vi "Collect Data.vi"(6 "Vicon Logging Signal":dbl, 7 "Motor Command":dbl, 8 "Current Time (s)":dbl, 9 "rt fifo":refnum<k33>, 10 "Target Lossy Data":T2, 11 "Sensors":T1) -> ()   [LabVIEW 2018]
uses:
  Target Lossy Data.ctl
  Sensor Data.ctl
  Target Logging Cluster.ctl
  Logging Data Cluster.ctl
  Target Logging Control Signals.ctl
  Target Logging Sensors.ctl
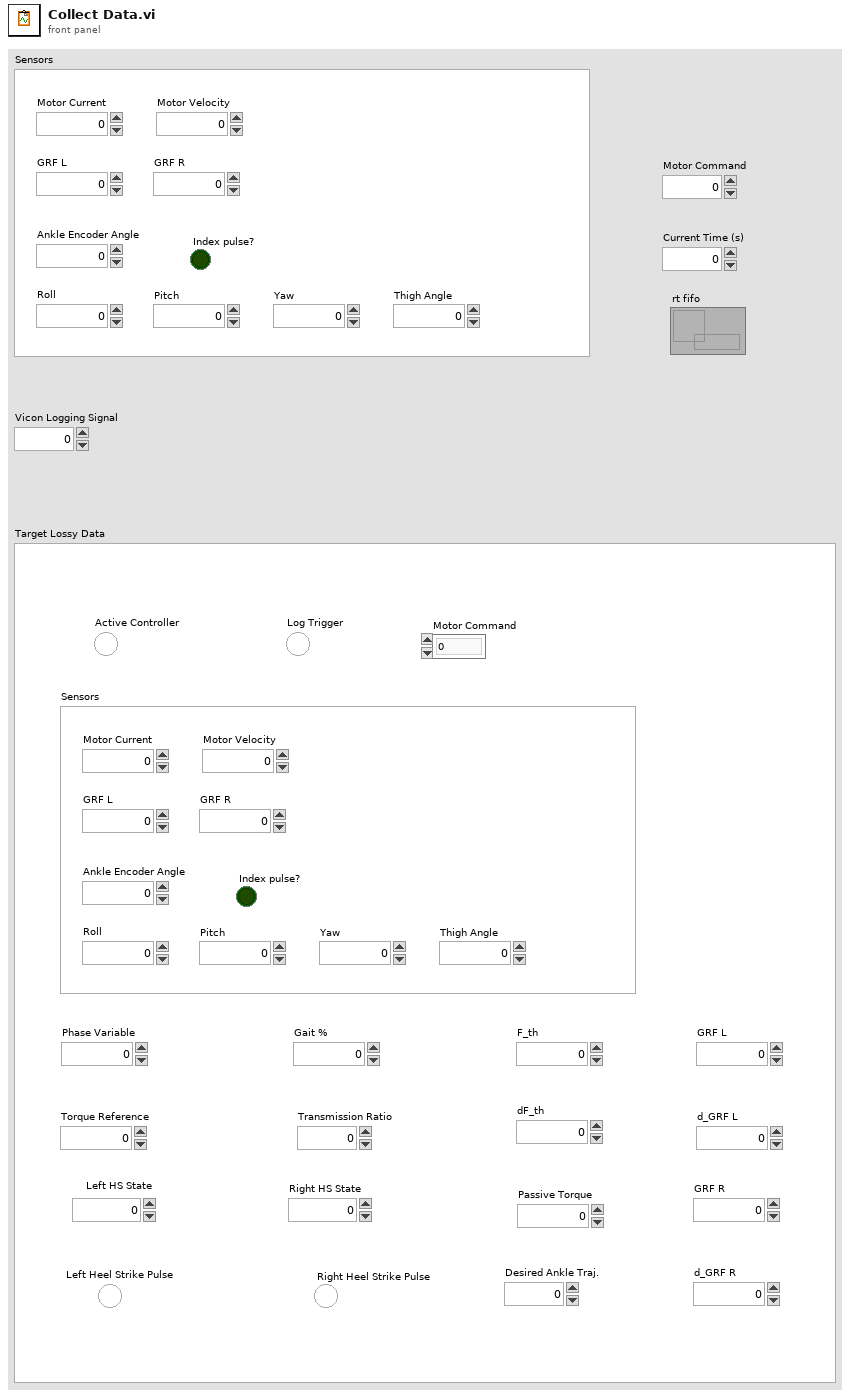
[diagram p1: front panel]
types:
  T1 = typedef "Sensor Data.ctl" = cluster{"Motor Current":dbl, "Motor Velocity":dbl, "Ankle Encoder Angle":dbl, "GRF L":dbl, "GRF R":dbl, "Index pulse?":bool, "Roll":dbl, "Pitch":dbl, "Yaw":dbl, "Thigh Angle":dbl}
  T2 = typedef "Target Lossy Data.ctl" = cluster{"Active Controller":bool, "Log Trigger":bool, "Sensors":T1, "Motor Command":dbl, "Phase Variable":dbl, "Left HS State":u32, "Left Heel Strike Pulse":bool, "Gait %":dbl, "Torque Reference":dbl, "Passive Torque":dbl, "F_th":dbl, "dF_th":dbl, "d_GRF L":dbl, "GRF L":dbl, "Transmission Ratio":dbl, "Desired Ankle Traj.":dbl, "Right HS State":u32, "Right Heel Strike Pulse":bool, "d_GRF R":dbl, "GRF R":dbl}
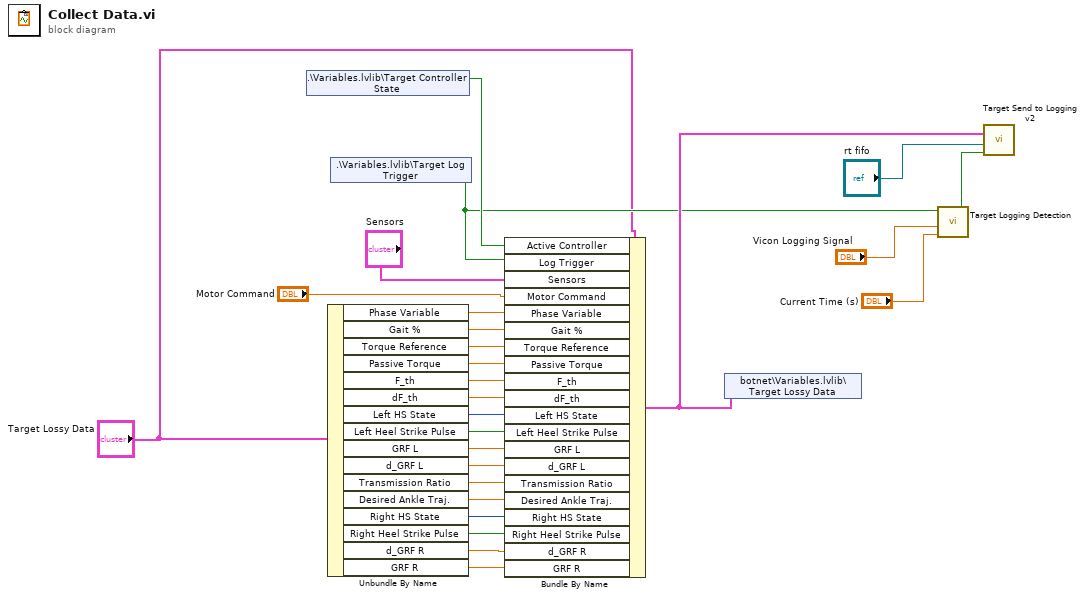
[diagram p0: block diagram]
diagram:
  n1 = shared-variable ".\\Variables.lvlib\\Target Controller State"() -> (w26:bool)  [unwired: 1 in, 1 out]
  n2 = Unbundle By Name("Target Lossy Data") -> ("Phase Variable"=w25:dbl, "Gait %"=w24:dbl, "Torque Reference"=w23:dbl, "Passive Torque"=w22:dbl, "F_th"=w21:dbl, "dF_th"=w20:dbl, "Left HS State"=w19:u32, "Left Heel Strike Pulse"=w18:bool, "GRF L"=w17:dbl, "d_GRF L"=w16:dbl, "Transmission Ratio"=w14:dbl, "Desired Ankle Traj."=w13:dbl, "Right HS State"=w5:u32, "Right Heel Strike Pulse"=w4:bool, "d_GRF R"=w3:dbl, "GRF R"=w2:dbl)
  n3 = shared-variable ".\\Variables.lvlib\\Target Log Trigger"() -> (w9:bool)  [unwired: 1 in, 1 out]
  n4 = Bundle By Name(cluster="Target Lossy Data", "Active Controller"=w26, "Log Trigger"=w9, "Sensors"="Sensors", "Motor Command"="Motor Command", "Phase Variable"=w25, "Gait %"=w24, "Torque Reference"=w23, "Passive Torque"=w22, "F_th"=w21, "dF_th"=w20, "Left HS State"=w19, "Left Heel Strike Pulse"=w18, "GRF L"=w17, "d_GRF L"=w16, "Transmission Ratio"=w14, "Desired Ankle Traj."=w13, "Right HS State"=w5, "Right Heel Strike Pulse"=w4, "d_GRF R"=w3, "GRF R"=w2) -> (w10:T2)
  n5 = shared-variable "botnet\\Variables.lvlib\\Target Lossy Data"(w10) -> ()  [unwired: 1 in, 1 out]
  n6 = call "Target Logging Detection.vi"("Main Clock Line (s)"="Current Time (s)", "Vicon Logging Signal"="Vicon Logging Signal", "Trigger High?"=w9) -> ("Valid for Logging?"=w12:bool)  [unwired: 8 in]
  n7 = call "Target Send to Logging v2.vi"("Valid for Logging or Not?"=w12, "rt fifo"="rt fifo", "Target Lossy Data"=w10) -> ()  [unwired: 9 in]
